vi "MAIN.vi"(8 "Error In":errorcluster) -> (0 "Error Out":errorcluster)   [LabVIEW 2019]
uses:
  analysis_main_states_enum_typedef.ctl
panel:
  in  "Stop":bool
  in  "Analyze Sample":bool
  in  "Setup Parameters":bool
  # "C-Axis Analysis"
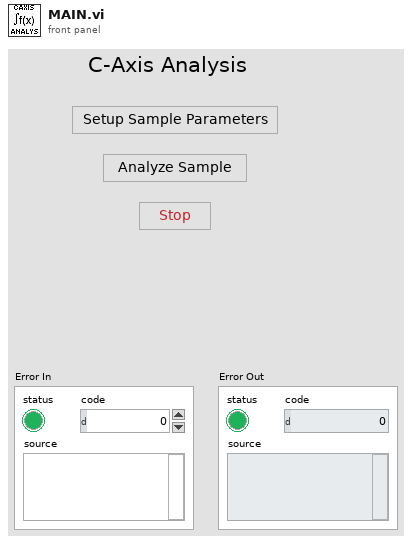
[diagram p1: front panel]
types:
  T1 = typedef "analysis_main_states_enum_typedef.ctl" = enum16{"Shutdown", "Analyze Sample", "Setup Parameters", "Wait", "Initialize"}
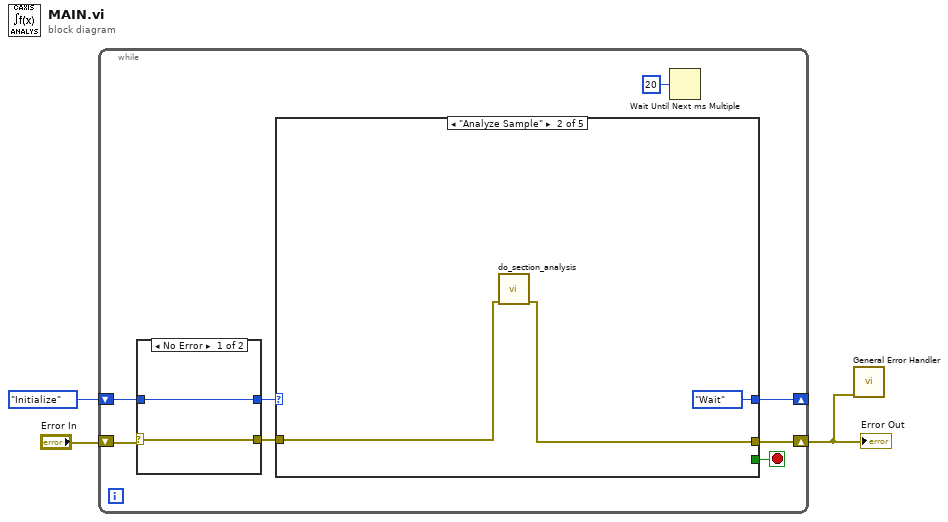
[diagram p0: block diagram]
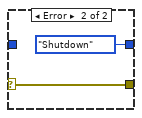
[diagram p2: hidden frame]
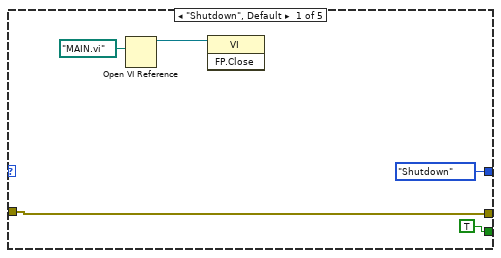
[diagram p3: hidden frame]
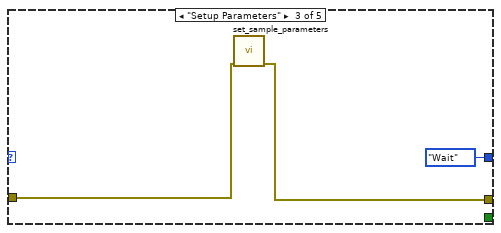
[diagram p4: hidden frame]
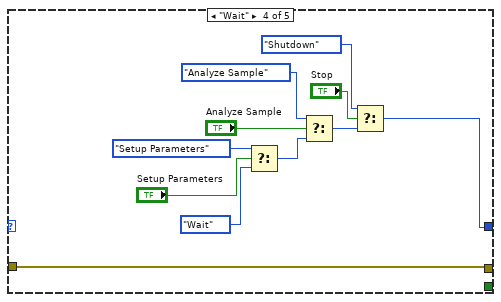
[diagram p5: hidden frame]
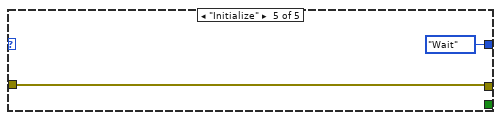
[diagram p6: hidden frame]
diagram:
  n1 = while {
    shift-right: [w5] -> _
    shift-left: analysis_main_states_enum_typedef."Initialize" -> [w8]
    shift-right: [w7] -> w1
    shift-left: "Error In" -> [w11]
    stop <- w6 stop-if-true
    n2 = case shown="No Error" w11 {
      selector: w11 -> [w13 w15]
      tunnel: [w13 w15] -> w10
      tunnel: [w12 analysis_main_states_enum_typedef."Shutdown"] -> w9
      tunnel: w8 -> [w12 _]
      frame No Error {
      }
      frame Error {
      }
    }
    n3 = case shown="\"Analyze Sample\"" w9 {
      tunnel: w10 -> [w20 w22 w25 w27 w38]
      tunnel: [w20 w21 w24 w27 w38] -> w7
      tunnel: [TRUE _ _ _ _] -> w6
      tunnel: [analysis_main_states_enum_typedef."Shutdown" analysis_main_states_enum_typedef."Wait" analysis_main_states_enum_typedef."Wait" w28 analysis_main_states_enum_typedef."Wait"] -> w5
      frame "Shutdown", Default {
        n4 = Open VI Reference(vi path=path "MAIN.vi") -> (vi reference=w16:refnum<vi>)  [unwired: 5 in, 1 out]
        n5 = invoke class="VI" method="FP.Close"(reference=w16) -> ()  [unwired: 2 in, 3 out]
      }
      frame "Analyze Sample" {
        n6 = call "do_section_analysis.vi"("Error In"=w22) -> ("Error Out"=w21:errorcluster)  [unwired: 10 in]
      }
      frame "Setup Parameters" {
        n7 = call "set_sample_parameters.vi"("Error In"=w25) -> ("Error Out"=w24:errorcluster)  [unwired: 10 in]
      }
      frame "Wait" {
        n8 = Select(t=analysis_main_states_enum_typedef."Setup Parameters", s="Setup Parameters", f=analysis_main_states_enum_typedef."Wait") -> (s? t:f=w36:T1)
        n9 = Select(t=analysis_main_states_enum_typedef."Analyze Sample", s="Analyze Sample", f=w36) -> (s? t:f=w37:T1)
        n10 = Select(t=analysis_main_states_enum_typedef."Shutdown", s="Stop", f=w37) -> (s? t:f=w28:T1)
      }
      frame "Initialize" {
      }
    }
    n11 = Wait Until Next ms Multiple(millisecond multiple=u32 20) -> ()  [unwired: 1 out]
  }
  "Error Out" <- w1
  n12 = call <vilib>:"General Error Handler.vi"("error in (no error)"=w1) -> ()  [unwired: 10 in, 5 out]
